vi "Call Palette View.vi"(9 "Theme Mode":u16(ring) items=["Light Theme", "Light Medium Contrast", "Light High Contrast", "Dark Theme", "Dark Medium Contrast", "Dark High Constrast"], 10 "VI ref in":refnum<vi>, 11 "Material Theme":refnum<class "Material Theme.lvclass">) -> (0 "error out":errorcluster, 2 "VI ref":refnum<vi>)   [LabVIEW 2021]
uses:
  Material-Scheme/Material-Scheme.lvclass
  Material Theme/Material Theme.lvclass
  Material-Scheme/View-User Colors.vi
  Theme Config.lvclass/Theme Config.ctl
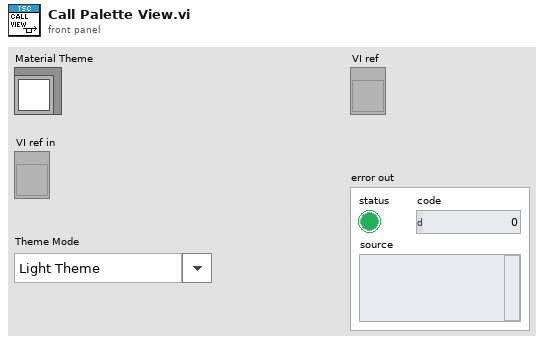
[diagram p1: front panel]
types:
  T1 = enum32{"Invalid", "Standard", "Closed", "Hidden", "Minimized", "Maximized"}
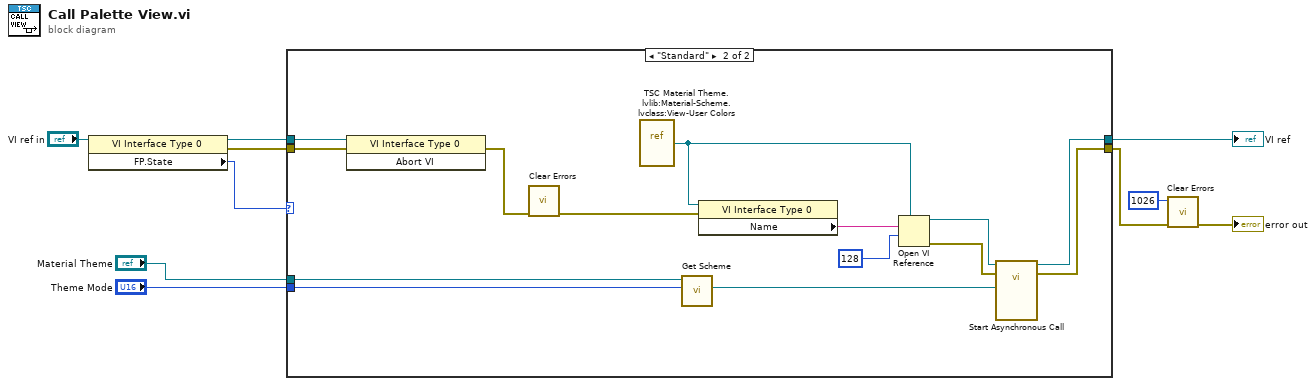
[diagram p0: block diagram]
diagram:
  n1 = property class="VI Interface Type 0"(reference="VI ref in") -> (reference out=w5:refnum<vi>, error out=w3:errorcluster, "FP.State"=w4:T1)  [unwired: 1 in]
  n2 = case shown="\"Standard\"" w4 {
    tunnel: "Material Theme" -> [_ w26]
    tunnel: "Theme Mode" -> [_ w25]
    tunnel: w5 -> [w12 w24]
    tunnel: [w12 w17] -> w7
    tunnel: [w11 w16] -> w6
    tunnel: w3 -> [w11 w13]
    frame Default {
    }
    frame "Standard" {
      n3 = invoke class="VI Interface Type 0" method="Abort VI"(reference=w24, error in=w13) -> (error out=w15:errorcluster)  [unwired: 1 in, 2 out]
      n4 = call <vilib>:"Clear Errors.vi"("error in (no error)"=w15) -> ("error out"=w14:errorcluster)  [unwired: 5 in, 1 out]
      n5 = vi-ref "TSC Material Theme.lvlib:Material-Scheme.lvclass:View-User Colors.vi"() -> (w19:refnum<vi>)
      n6 = call "Get Scheme.vi"("Theme"=w25, "Material Theme in"=w26) -> ("Material-Scheme"=w23:refnum<class "Material-Scheme.lvclass">)  [unwired: 7 in, 2 out]
      n7 = property class="VI Interface Type 0"(reference=w19, error in=w14) -> ("Name"=w22:string)  [unwired: 2 out]
      n8 = Open VI Reference(type specifier VI Refnum (for type only)=w19, vi path=w22, options=128) -> (vi reference=w20:refnum<vi>, error out=w18:errorcluster)  [unwired: 3 in]
      n9 = call-by-ref "Start Asynchronous Call"(reference=w20, error in=w18, "Material-Scheme.lvclass"=w23) -> (reference out=w17:refnum<vi>, error out=w16:errorcluster)  [unwired: 11 in]
    }
  }
  "VI ref" <- w7
  n10 = call <vilib>:"Clear Errors.vi"("error in (no error)"=w6, "specific error code to clear (0: all)"=1026) -> ("error out"=→"error out":errorcluster)  [unwired: 4 in, 1 out]
